vi "Compile Asynchronous Execution Units.vi"(0 "Device Ref in":T3=18446744073709551615 format="%.0x", 1 "Asynchronous Execution Units":cluster{"Grouped Execution Units":T4[]}[](array[cluster]) {"Grouped Execution Units"."ReadWrite Channels" format="%.0x"; "Grouped Execution Units"."Outgoing Channels" format="%.0x"; "Grouped Execution Units"."Incoming Channels" format="%.0x"}, 3 "error in":errorcluster) -> (7 "Device Ref out":T3=18446744073709551615 format="%.0x", 8 "Compiled Asynchronous Execution Units":T2(array[cluster]), 10 "error out":errorcluster)   [LabVIEW 2020, in "Ballard MIL-STD-1553 System Explorer.lvlib"]
uses:
  Ballard MIL-STD-1553 System Explorer.lvlib
  Includes/Ballard MIL-STD-1553 Engine.lvlibp/Engine/Interfaces/Controls/Execution Unit Information.ctl
  Includes/Ballard MIL-STD-1553 Engine.lvlibp/Engine/Interfaces/Execution Unit/Execution Unit.lvclass
  Includes/Ballard MIL-STD-1553 Engine.lvlibp/1abvi3w/vi.lib/NI VeriStand/Custom Device API/Custom Device Item Ref.ctl
  <vilib>/NI VeriStand/Custom Device API/Custom Device Item Ref.ctl
  Shared/Asynchronous Execution Unit Compiled Information.ctl
  <vilib>/NI VeriStand/Custom Device API/Custom Device API.lvlib
  <vilib>/NI/NIVS Inline Async API/_Data Access System Explorer/Data Access System Explorer.lvlib
  Shared/Ballard MIL-STD-1553 Shared.lvlib
  Includes/Ballard MIL-STD-1553 Engine.lvlibp/Engine/Interfaces/Interfaces.lvlib
  Includes/Ballard MIL-STD-1553 Engine.lvlibp/1abvi3w/vi.lib/NI VeriStand/Custom Device API/Custom Device API.lvlib
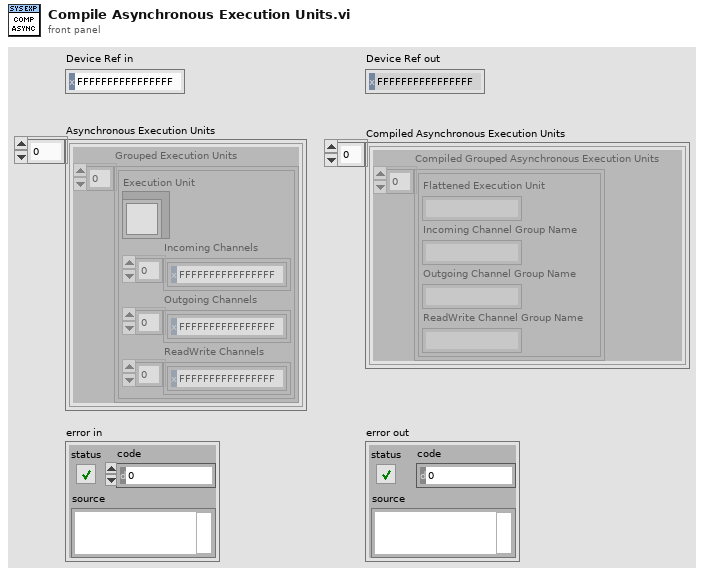
[diagram p1: front panel]
types:
  T1 = typedef "Ballard MIL-STD-1553 Shared.lvlib/Asynchronous Execution Unit Compiled Information.ctl" = cluster{"Flattened Execution Unit":string, "Incoming Channel Group Name":string, "Outgoing Channel Group Name":string, "ReadWrite Channel Group Name":string}
  T2 = cluster{"Compiled Grouped Asynchronous Execution Units":T1[]}[]
  T3 = typedef "Custom Device API.lvlib/Custom Device Item Ref.ctl" = u64
  T4 = typedef "Ballard MIL-STD-1553 Engine.lvlibp/Interfaces.lvlib/Execution Unit Information.ctl" = cluster{"Execution Unit":refnum<class "Execution Unit.lvclass">, "Incoming Channels":T5[], "Outgoing Channels":T5[], "ReadWrite Channels":T5[]}
  T5 = typedef "Ballard MIL-STD-1553 Engine.lvlibp/Custom Device API.lvlib/Custom Device Item Ref.ctl" = u64
  T6 = enum16{"Output/Write", "Input/Read", "Input/ReadWrite"}
  T7 = cluster{"Name":string, "Type":enum16{"Output/Write", "Input/Read", "Input/ReadWrite"}, "VS Refs":T3[]}
  T8 = cluster{"Name":string, "Type":enum16{"Output/Write", "Input/Read", "Input/ReadWrite"}, "VS Refs":T3[]}[]
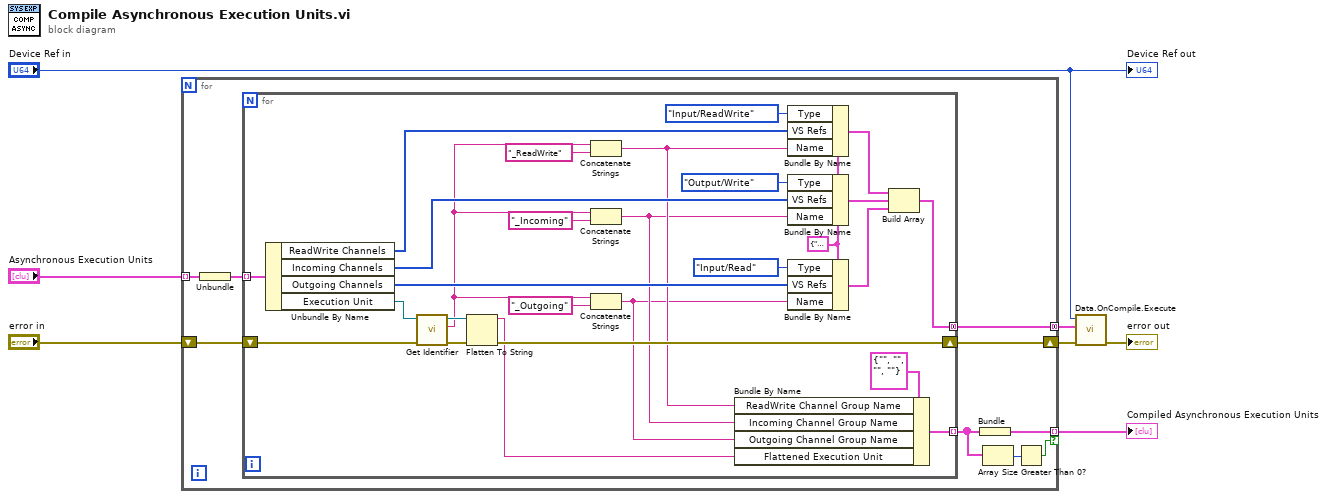
[diagram p0: block diagram]
diagram:
  n1 = for {
    tunnel: "Asynchronous Execution Units" -> [w16] mode=indexing
    tunnel: [w15] -> w6 mode=concatenating
    tunnel: [w11] -> w1 mode=indexing if=w8
    shift-right: [w13] -> w2
    shift-left: "error in" -> [w14]
    n2 = Unbundle(w16) -> ("Grouped Execution Units"=w12:T4[])
    n3 = for {
      tunnel: w12 -> [w42] mode=indexing
      tunnel: [w35] -> w15 mode=concatenating
      shift-right: [w34] -> w13
      shift-left: w14 -> [w33]
      tunnel: [w28] -> w10 mode=indexing
      w26 = T7 {"Name"="", "Type"=enum."Output/Write", "VS Refs"=[]} ("Group")
      n4 = Unbundle By Name(w42) -> ("ReadWrite Channels"=w24:T5[], "Incoming Channels"=w43:T5[], "Outgoing Channels"=w37:T5[], "Execution Unit"=w31:refnum<class "Execution Unit.lvclass">)
      n5 = call-dynamic "Get Identifier.vi"("error in (no error)"=w33, "Execution Unit in"=w31) -> ("error out"=w32:errorcluster, "Identifier"=w22:string, "Execution Unit out"=w30:refnum<class "Execution Unit.lvclass">)  [unwired: 7 in]
      n6 = Flatten To String(anything=w30, error in (no error)=w32) -> (data string=w21:string, error out=w34:errorcluster)  [unwired: 2 in, 1 out]
      n7 = Concatenate Strings(w22, "_ReadWrite" ("string")) -> (w19:string)
      n8 = Concatenate Strings(w22, "_Incoming" ("string")) -> (w18:string)
      n9 = Concatenate Strings(w22, "_Outgoing" ("string")) -> (w17:string)
      n10 = Bundle By Name(cluster=T1 {"Flattened Execution Unit"="", "Incoming Channel Group Name"="", "Outgoing Channel Group Name"="", "ReadWrite Channel Group Name"=""} ("Asynchronous Execution Unit Compiled Information"), "ReadWrite Channel Group Name"=w19, "Incoming Channel Group Name"=w18, "Outgoing Channel Group Name"=w17, "Flattened Execution Unit"=w21) -> (w28:T1)
      n11 = Bundle By Name(cluster=w26, "Type"=T6."Input/ReadWrite", "VS Refs"=w24, "Name"=w19) -> (w20:T7)
      n12 = Bundle By Name(cluster=w26, "Type"=T6."Output/Write", "VS Refs"=w43, "Name"=w18) -> (w27:T7)
      n13 = Bundle By Name(cluster=w26, "Type"=T6."Input/Read", "VS Refs"=w37, "Name"=w17) -> (w36:T7)
      n14 = Build Array(w20, w27, w36) -> (w35:T8)
    }
    n15 = Bundle(w10) -> (w11:cluster{T1[]})  [unwired: 1 in]
    n16 = Array Size(array=w10) -> (size(s)=w9:i32)
    n17 = Greater Than 0?(x=w9) -> (x > 0?=w8:bool)
  }
  "Compiled Asynchronous Execution Units" <- w1
  n18 = call <vilib>:"Data.OnCompile.Execute.vi"("error in"=w2, "VS Ref Groups"=w6, "Custom Device Ref"="Device Ref in") -> ("error out"=→"error out":errorcluster)  [unwired: 7 in, 1 out]
  "Device Ref out" <- "Device Ref in"
